vi "Get ClientID from Session.vi"(8 "error in (no error)":errorcluster, 10 "SessionMailbox":refnum<queue>, 11 "MQTT Server":refnum<class "Server.lvclass">) -> (0 "error out":errorcluster, 1 "found?":bool, 2 "Client ID":string, 3 "MQTT Server":refnum<class "Server.lvclass">)   [LabVIEW 2013, in "MQTT Server.lvlib" / "Server.lvclass"]
uses:
  Server.lvclass
  <vilib>/LabVIEW Open Source Project/MQTT Connection/MQTT_Base/Base Class/Response -- cluster.ctl
  <vilib>/LabVIEW Open Source Project/MQTT Control Packets/Control Packets/ControlPacket/ControlPacket.lvclass
  Server.lvclass/Server.ctl
  <vilib>/LabVIEW Open Source Project/MQTT Connection/MQTT_Base/Base Class/MQTT_Base.lvclass
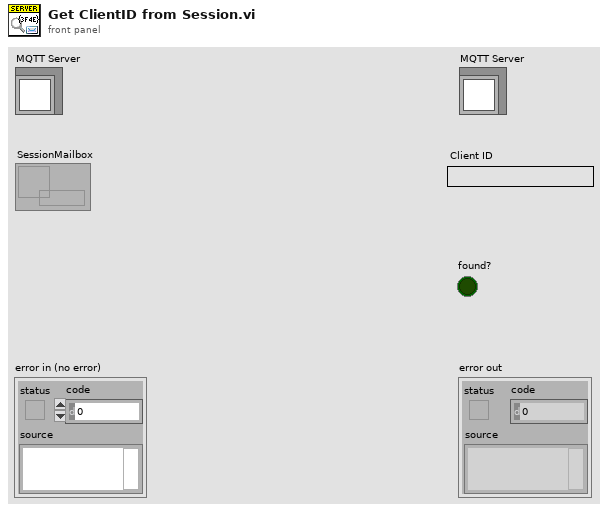
[diagram p1: front panel]
types:
  T1 = typedef "MQTT Server.lvlib/Server.lvclass/SessionRef -- cluster.ctl" = cluster{"ClientID":string, "SessionMailbox":refnum<queue>}
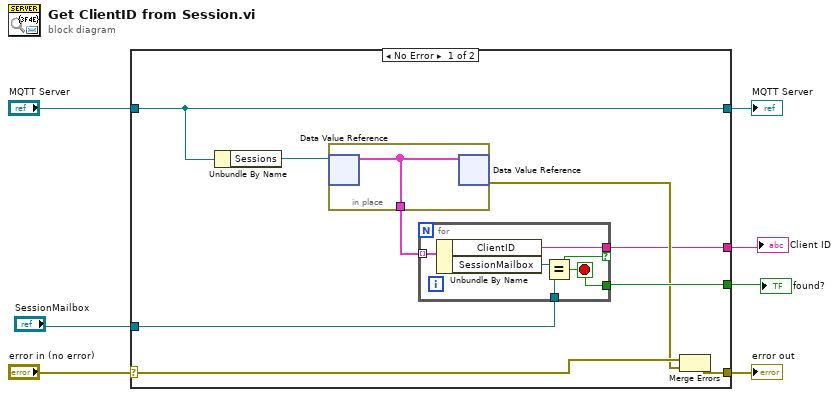
[diagram p0: block diagram]
diagram:
  n1 = case shown="No Error" "error in (no error)" {
    selector: "error in (no error)" -> [w12 w24]
    tunnel: [w10 w24] -> w6
    tunnel: [w16 w23] -> w4
    tunnel: "MQTT Server" -> [w16 w23]
    tunnel: "SessionMailbox" -> [w9 _]
    tunnel: [w13 _] -> w2
    tunnel: [w8 _] -> w1
    frame No Error {
      n2 = Unbundle By Name(w16) -> ("Sessions"=w15:refnum<data-value>)
      n3 = in-place {
        in-place-border: [w22] -> w14
        n4 = in-place-dvr #1(w15) -> (w22:T1[])  [unwired: 1 out]
        n5 = in-place-dvr #1(w22) -> (w11:errorcluster)  [unwired: 1 out]
      }
      n6 = for {
        tunnel: w14 -> [w21] mode=indexing
        tunnel: w9 -> [w19]
        tunnel: [w18] -> w8 if=w17
        tunnel: [w17] -> w13
        stop <- w17 stop-if-true
        n7 = Unbundle By Name(w21) -> ("ClientID"=w18:string, "SessionMailbox"=w20:refnum<queue>)
        n8 = Equal?(x=w20, y=w19) -> (x = y?=w17:bool)
      }
      n9 = Merge Errors(w12, w11) -> (w10:errorcluster)
    }
    frame Error {
    }
  }
  "error out" <- w6
  "MQTT Server" <- w4
  "found?" <- w2
  "Client ID" <- w1
